vi "Create Session.vi"(8 "error in (no error)":errorcluster, 10 "TS License Type":T1, 11 "Dev Debug?":bool) -> (0 "error out":errorcluster, 3 "Engine out":refnum<class "Engine.lvclass">)   [LabVIEW 2020, in "TSnax.lvlib" / "Engine.lvclass"]
uses:
  Engine.lvclass
  TS License Type.ctl
  Engine.lvclass/Engine.ctl
  Session Daemon Async.vi
  TSnax.lvlib
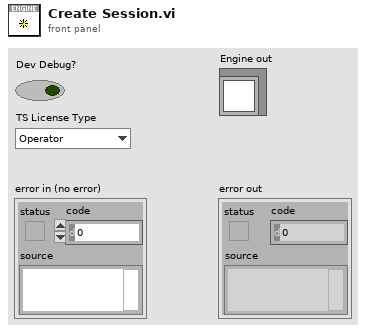
[diagram p1: front panel]
types:
  T1 = typedef "TSnax.lvlib/TS License Type.ctl" = enum16{"Operator", "CustomEditor", "SequenceEditor"}
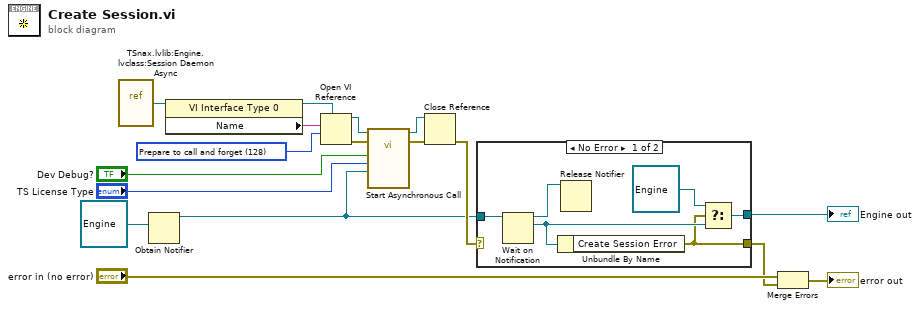
[diagram p0: block diagram]
diagram:
  w10 = 128 items=["Record modifications"=1, "Open templates for editing"=2, "Prompt user to save"=4, "Prepare for reentrant run"=8, "Prompt to find missing subVIs"=16, "Hide loading dialog box"=32, "Enable simultaneous calls"=64, "Prepare to call and forget"=128, "Simultaneous call and forget"=192, "Prepare to call and collect"=256, "Simultaneous call and collect"=320]
  n1 = vi-ref "TSnax.lvlib:Engine.lvclass:Session Daemon Async.vi"() -> (w8:refnum<vi>)
  n2 = Obtain Notifier(notification data type=refnum<class "Engine.lvclass"> refnum ("TSnax.lvlib:Engine.lvclass")) -> (notifier out=w4:refnum<notifier>)  [unwired: 3 in, 2 out]
  n3 = property class="VI Interface Type 0"(reference=w8) -> (reference out=w11:refnum<vi>, "Name"=w9:string)  [unwired: 1 in, 1 out]
  n4 = Open VI Reference(type specifier VI Refnum (for type only)=w11, vi path=w9, options=w10) -> (vi reference=w13:refnum<vi>, error out=w12:errorcluster)  [unwired: 3 in]
  n5 = call-by-ref "Start Asynchronous Call"(reference=w13, error in=w12, "Engine Notifier"=w4, "TS License Type"="TS License Type", "Dev Debug?"="Dev Debug?") -> (reference out=w15:refnum<vi>, error out=w14:errorcluster)  [unwired: 9 in]
  n6 = Close Reference(reference=w15, error in (no error)=w14) -> (error out=w17:errorcluster)
  n7 = case shown="No Error" w17 {
    selector: w17 -> [_ w24]
    tunnel: w4 -> [w23 _]
    tunnel: [w19 _] -> w3
    tunnel: [w18 w24] -> w1
    frame No Error {
      n8 = Wait on Notification(notifier=w23) -> (notifier out=w22:refnum<notifier>, notification=w21:refnum<class "Engine.lvclass">)  [unwired: 3 in, 2 out]
      n9 = Unbundle By Name(w21) -> ("Create Session Error"=w18:errorcluster)
      n10 = Release Notifier(notifier=w22) -> ()  [unwired: 2 in, 3 out]
      n11 = Select(t=refnum<class "Engine.lvclass"> refnum, s=w18, f=w21) -> (s? t:f=w19:refnum<class "Engine.lvclass">)
    }
    frame Error {
    }
  }
  "Engine out" <- w3
  n12 = Merge Errors("error in (no error)", w1) -> (→"error out":errorcluster)
